vi "Programmatically Run Tests from File.vi"   [LabVIEW 2023]
doc: "Demonstrates how to use the LabVIEW Unit Test Framework Toolkit to execute tests from test files programmatically."
uses:
  <vilib>/utf/dialogs/utf_testsuite_report_type.ctl
  <vilib>/utf/NI_UnitTestFramework.lvlib
panel:
  # "Overview: Demonstrates how to use the Unit Test Framework Toolkit to execute tests from test files programmatically.\nRequirements: LabVIEW Full Development System, Unit Test Framework Toolkit\nInstructions:\n1.  Display the block diagram by selecting Windows>>Show Block Diagram.\n2.  Specify the directory which contains the test files you want to execute in the test file path path constant. This VI sets the labview\\examples\\Unit Test Framework\\Basic Functions directory as default. Make sure the folder you specified and this VI are in the same directory so that you do not need to change the relative path.\n3. Run this VI. The Unit Test Framework Toolkit displays the Unit Test Framework Results window and a report after test execution."
types:
  T1 = typedef "NI_UnitTestFramework.lvlib/utf_testsuite_report_type.ctl" = u16
  T2 = typedef "NI_UnitTestFramework.lvlib/utf_test_result_overall.ctl" = cluster{"utf results out":T3[], "untested VIs":cluster{"VI path":path, "code coverage":T12, "vi hierarchy":string[]}[], "project file path":path, "system information":string}
  T3 = typedef "NI_UnitTestFramework.lvlib/utf_test_result_testfile.ctl" = cluster{"test case":T4[], "test status":T5, "test path":path, "setup VI":path, "teardown VI":path, "code coverage":T12, "start time":timestamp, "end time":timestamp, "test hierarchy":string[], "VI path":path, "VI timestamp":timestamp, "VI rev hist":i32, "requirements ID":string, "array brackets":string, "name separator":string, "errors":T13[], "paragraph header":string, "result comment":string, "vi hierarchy":string[], "subVI coverage info":T12[], "subVI info":T15[], "big array threshold":u32, "VI Index":i32, "Comment":string, "Dynamic Dispatch":bool, "User-defined test VI":path, "user-defined VI code coverage":T12}
  T4 = typedef "NI_UnitTestFramework.lvlib/utf_test_result_testcase.ctl" = cluster{"test result":T5, "run Times":T6[], "test case name":string, "requirements":string, "code coverage":T12, "subVI coverage info":T12[]}
  T5 = typedef "NI_UnitTestFramework.lvlib/utf_test_result.ctl" = enum16{"Passed", "Failed", "Error", "Skipped", "Not Processed"}
  T6 = typedef "NI_UnitTestFramework.lvlib/utf_test_result_troll_new.ctl" = cluster{"result (test)":T5, "Vector Result":T7[]}
  T7 = typedef "NI_UnitTestFramework.lvlib/utf_vector_result.ctl" = cluster{"time elapsed [ms]":u32, "result (test)":T5, "result (parameters)":T8[], "Used Vector Values":cluster{"Vector Name":string, "element":i32}[], "Executed Class Path":path, "Input":T11[]}
  T8 = typedef "NI_UnitTestFramework.lvlib/utf_test_result_failure.ctl" = cluster{"result":T5, "error message":string, "parameter name":string, "parameter value":variant, "parameters":variant[], "comparison":T9, "requirement ID":string, "VI":T10, "Used Vector Name":string}
  T9 = typedef "NI_UnitTestFramework.lvlib/utf_test_comparison_operators.ctl" = enum16{"=", "!=", ">", ">=", "<", "<=", "range", "symmetric tolerance", "asymmetric tolerance", "string contains", "string not contain", "array size", "string length", "array range", "by element", "array range (limit array)", "user-defined", "array contains", "array not contain", "vector length", "= (elm)", "!= (elm)", "= (case insensitive)", "!= (case insensitive)"}
  T10 = typedef "NI_UnitTestFramework.lvlib/utf_vi_tag.ctl" = enum16{"Setup VI", "VI under Test", "Teardown VI"}
  T11 = typedef "NI_UnitTestFramework.lvlib/utf_test_result_input_data.ctl" = cluster{"Name":string, "Input Value":variant[], "VI":T10, "Used Vector Index":i32}
  T12 = typedef "NI_UnitTestFramework.lvlib/utf_code_coverage.ctl" = cluster{"coverage":dbl, "diagram run flag":bool[]}
  T13 = typedef "NI_UnitTestFramework.lvlib/utf_error_data.ctl" = cluster{"error type":T14, "description":string}
  T14 = typedef "NI_UnitTestFramework.lvlib/utf_error_type.ctl" = enum16{"TestFileError", "VIError", "SetupVIError", "TearDownVIError", "OtherError"}
  T15 = typedef "NI_UnitTestFramework.lvlib/utf_subvi_info.ctl" = cluster{"Path":path, "Dependence VI":bool}
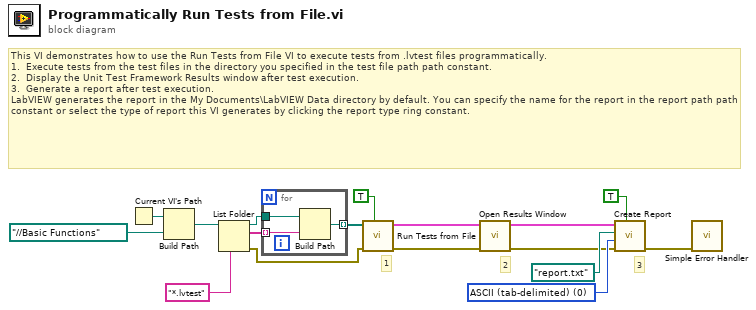
[diagram p0: block diagram]
diagram:
  w12 = T1 0 items=["ASCII (tab-delimited)", "HTML", "ATML (XML-based)"] ("report type")
  # "3"
  # "2"
  # "1"
  # "This VI demonstrates how to use the Run Tests from File VI to execute tests from .lvtest files programmatically.\n1.  Execute tests from the test files in the directory you specified in the test file path path constant.\n2.  Display the Unit Test Framework Results window after test execution.\n3.  Generate a report after test execution.\nLabVIEW generates the report in the My Documents\\LabVIEW Data directory by default. You can specify the name for the report in the report path path constant or select the type of report this VI generates by clicking the report type ring constant."
  n1 = Current VI's Path() -> (path=w3:path)
  n2 = Build Path(base path=w3, name or relative path=path "../../Basic Functions" ("project file path")) -> (appended path=w7:path)
  n3 = List Folder(path=w7, pattern="*.lvtest") -> (path out=w1:path, filenames=w8:string[], error out=w2:errorcluster)  [unwired: 1 in, 2 out]
  n4 = for {
    tunnel: w8 -> [w20] mode=indexing
    tunnel: w1 -> [w19]
    tunnel: [w18] -> w6 mode=indexing
    n5 = Build Path(base path=w19, name or relative path=w20) -> (appended path=w18:path)
  }
  n6 = call <vilib>:"Run Tests from File.vi"("show progress bar? (T)"=TRUE ("show progress bar"), "error in (no error)"=w2, "test file paths"=w6) -> ("error out"=w15:errorcluster, "test results out"=w10:T2)  [unwired: 7 out]
  n7 = call <vilib>:"Open Results Window.vi"("error in (no error)"=w15, "test results in"=w10) -> ("error out"=w11:errorcluster, "test results out"=w9:T2)  [unwired: 8 out]
  n8 = call <vilib>:"Create Report.vi"("view report? (T)"=TRUE ("view report"), "error in (no error)"=w11, "report type (HTML)"=w12, "report path"=path "report.txt", "test results in"=w9) -> ("error out"=w5:errorcluster)  [unwired: 3 in, 3 out]
  n9 = call <vilib>:"Simple Error Handler.vi"("error in (no error)"=w5) -> ()  [unwired: 1 in, 8 out]
